vi "Scripting Example.vi"() -> ()   [LabVIEW 2019]
uses:
  NationalInstruments.VeriStand.SystemDefinitionAPI
  <vilib>/NI VeriStand/Custom Device API/Custom Device Item Ref.ctl
  Scripting API/Polymorphic/Create Message_TriggerOnly.vi
  Scripting API/Polymorphic/Add Response_Wait sec.vi
  Addon/Support Libraries/Protocols.lvlibp/TCP/TCP.lvclass
  Scripting API/Scripting API.lvlib
  <vilib>/NI VeriStand/Custom Device API/Custom Device API.lvlib
panel:
  in  "Exported File path":path
  out "error out":errorcluster
  in  "Target in":refnum<k24>
  in  "error in":errorcluster
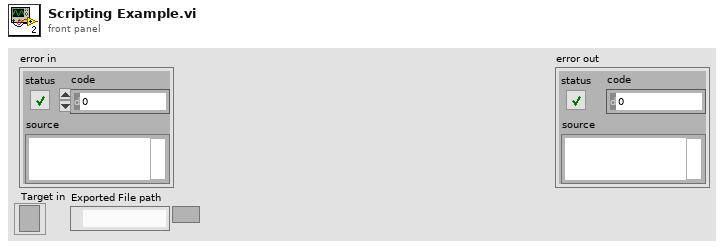
[diagram p1: front panel]
types:
  T1 = typedef "Custom Device API.lvlib/Custom Device Item Ref.ctl" = u64
  T2 = cluster{"Response":string, "Linkages":cluster{"Variable name":string, "Linked Channel refnum":T1}[], "Wait value":dbl, "Use Byte Count channel?":bool, "Channel refnum":T1}
  T3 = cluster{"Command":string, "Linkages":cluster{"Variable name":string, "Linked Channel refnum":T1}[], "Use Padding?":bool, "Padding":cluster{"Length":u16, "Pad Value":u16}}
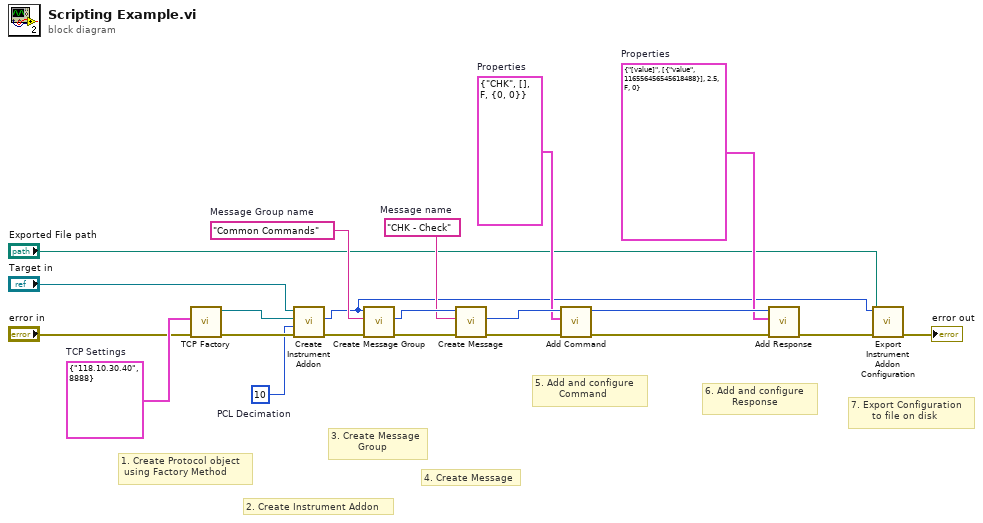
[diagram p0: block diagram]
diagram:
  w5 = T2 {"Response"="[value]", "Linkages"=[{"Variable name"="value", "Linked Channel refnum"=116556456545618488}], "Wait value"=2.5, "Use Byte Count channel?"=FALSE, "Channel refnum"=0}  # Properties
  w8 = T3 {"Command"="CHK", "Linkages"=[], "Use Padding?"=FALSE, "Padding"={"Length"=0, "Pad Value"=0}}  # Properties
  w11 = "CHK - Check"  # Message name
  w14 = "Common Commands"  # Message Group name
  w19 = u16 10  # PCL Decimation
  w21 = cluster{"IP Address":string, "Port":u16} {"IP Address"="118.10.30.40", "Port"=8888}  # TCP Settings
  # "7. Export Configuration\n       to file on disk"
  # "6. Add and configure\n         Response"
  # "5. Add and configure\n        Command"
  # "4. Create Message"
  # "3. Create Message\n         Group"
  # "2. Create Instrument Addon"
  # "1. Create Protocol object\n using Factory Method"
  n1 = call "TCP Factory.vi"("error in (no error)"="error in", "TCP Settings"=w21) -> ("error out"=w20:errorcluster, "TCP out"=w18:refnum<class "TCP.lvclass">)  [unwired: 8 in]
  n2 = call "Create Instrument Addon.vi"("error in (no error)"=w20, "PCL Decimation"=w19, "Protocol in"=w18, "Target in"="Target in") -> ("error out"=w15:errorcluster, "Instrument Addon Custom Device refnum"=w4:T1)  [unwired: 4 in, 2 out]
  n3 = call "Create Message Group.vi"("error in (no error)"=w15, "Message Group name"=w14, "Instrument Addon refnum in"=w4) -> ("error out"=w12:errorcluster, "Message Group refnum out"=w13:T1)  [unwired: 6 in, 1 out]
  n4 = call-poly "Create Message.vi"("error in (no error)"=w12, "Message name"=w11, "Message Group refnum in"=w13) -> ("error out"=w10:errorcluster, "Message refnum out"=w9:T1)  [unwired: 6 in, 1 out]
  n5 = call "Add Command.vi"("error in (no error)"=w10, "Settings"=w8, "Message refnum in"=w9) -> ("error out"=w7:errorcluster, "Message refnum out"=w6:T1)  [unwired: 6 in, 1 out]
  n6 = call-poly "Add Response.vi"("error in (no error)"=w7, "Settings"=w5, "Response refnum in"=w6) -> ("error out"=w3:errorcluster)  [unwired: 7 in, 1 out]
  n7 = call "Export Instrument Addon Configuration.vi"("error in (no error)"=w3, "Exported File path"="Exported File path", "Instrument Addon refnum in"=w4) -> ("error out"=→"error out":errorcluster)  [unwired: 7 in, 1 out]
